vi "xyz_llh_converter.vi"() -> ()   [LabVIEW 2020]
uses:
  GPS_SIM_CREATE_BIN.dll
panel:
  out "xyz":dbl[](array[numeric]) format="%#.6g"
  out "z":dbl format="%#.6g"
  out "y":dbl format="%#.6g"
  out "x":dbl format="%.6g"
  in  "height":dbl=100.0
  in  "lon":dbl=120.032669
  in  "lat":dbl=30.286502
  out "error out":errorcluster
  # "30.286502, 120.032669, 100"
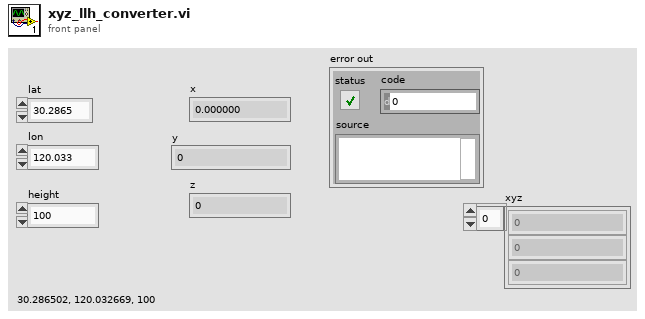
[diagram p1: front panel]
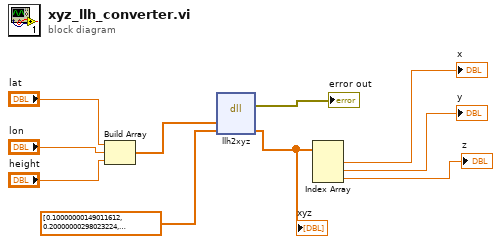
[diagram p0: block diagram]
diagram:
  n1 = Build Array("lat", "lon", "height") -> (w6:dbl[])
  n2 = dll-call lib="PTH2iabs CUsersduygaOneDriveデスクトップWORKS\nNissan GPS\tbuild dllGPS_SIM_CREATE_BIN.dll" fn="llh2xyz"("llh"=w6, "xyz"=dbl[] [0.10000000149011612, 0.20000000298023224, 10.300000190734863] ("appended array")) -> (error out=→"error out":errorcluster, "xyz"=w5:dbl[])  [unwired: 5 in, 1 out]
  "xyz" <- w5
  n3 = Index Array(array=w5) -> (element #1=→"x":dbl, element #2=→"y":dbl, element #3=→"z":dbl)  [unwired: 3 in]
